vi "Simulate1.vi"() -> ()   [LabVIEW 2014, in "MyHostCode.lvlib"]
uses:
  MyHostCode.lvlib
  FPGACode/Lead Enum.ctl
  <vilib>/Utility/file.llb/Read From Spreadsheet File (DBL).vi
  <vilib>/FPGAPlugInAG/USB-7856R/niLvFpga_Open_USB-7856R.vi
  <vilib>/rvi/interface/common/dynamic/niFpgaDynamicAddResources.vi
  <vilib>/FPGAPlugInAG/Dynamic/niLvFpga_Reset_Dynamic.vi
  <vilib>/FPGAPlugInAG/Dynamic/niLvFpga_Run_Dynamic.vi
  <vilib>/Utility/error.llb/Error Cluster From Error Code.vi
  <vilib>/rvi/errors/niLvFpgaAdjustHostInterfaceError.vi
  <vilib>/FPGAPlugInAG/Dynamic/niLvFpga_Close_Dynamic.vi
  <vilib>/rvi/interface/nirviOpenFPGA/nirviOpenFPGA.xnode
  FPGA Bitfiles/ECGPWMAdaptiveFi_FPGATarget2_ECGAFsim_UMxt-cFiVhs.lvbitx
  <vilib>/rvi/interface/nirviMethod/nirviMethod.xnode
  <vilib>/rvi/interface/nirviReadWriteControl/nirviReadWriteControl.xnode
  <vilib>/rvi/interface/nirviCloseFPGA/nirviCloseFPGA.xnode
  <vilib>/rvi/errors/niLvFpgaMergeErrorWithErrorCode.vi
  <vilib>/FPGAPlugInAG/Dynamic/niLvFpga_StartFifo_Dynamic.vi
  <vilib>/FPGAPlugInAG/Dynamic/niLvFpga_ReadFifo_Dynamic.vi
  <vilib>/rvi/interface/Simulation/niFpgaSimulationCallBeginRW.vi
  NiFpgaLv.dll
  <vilib>/FPGAPlugInAG/Dynamic/niLvFpga_WriteFifo_Dynamic.vi
panel:
  out "Waveform Chart":dbl[](graph)
  out "Waveform Graph 2":dbl[](graph)
  out "Waveform Graph":dbl[](graph)
  out "Data":fxp<+/-,32,16>[](array[numeric]) format="%.21g"
  out "Number":u32
  out "# elements in queue 2":i32
  in  "Reset":bool
  in  "stop":bool
  out "WeightSum":fxp<+/-,33,19> format="%.20g"
  out "BetaProduct":fxp<+/-,32,-1> format="%.33g"
  in  "Rescale":bool
  in  "Decimate":bool
  out "ECG":i16[][](graph)
  out "Gradients":i16[][](graph)
  out "Invasive Blood Pressure":i16[][](graph)
  in  "Plot Info":T2={"Element"={"Lead"=enum."RA", "Filter"=TRUE}, "Element 2"={"Lead"=enum."LA", "Filter"=TRUE}, "Element 3"={"Lead"=enum."LL", "Filter"=TRUE}, "Element 4"={"Lead"=enum."V1", "Filter"=TRUE}, "Element 5"={"Lead"=enum."V2", "Filter"=TRUE}, "Element 6"={"Lead"=enum."V3", "Filter"=TRUE}, "Element 7"={"Lead"=enum."I", "Filter"=TRUE}, "Element 8"={"Lead"=enum."II", "Filter"=TRUE}}
  out "# elements in queue":i32
  in  "File Path Control":path=path "C:/Users/pursley/Documents/Projects/NHLBI/Lederman/Testing/2014-03-21/FL1.txt"
  in  "Beta":fxp<+/-,32,-16>
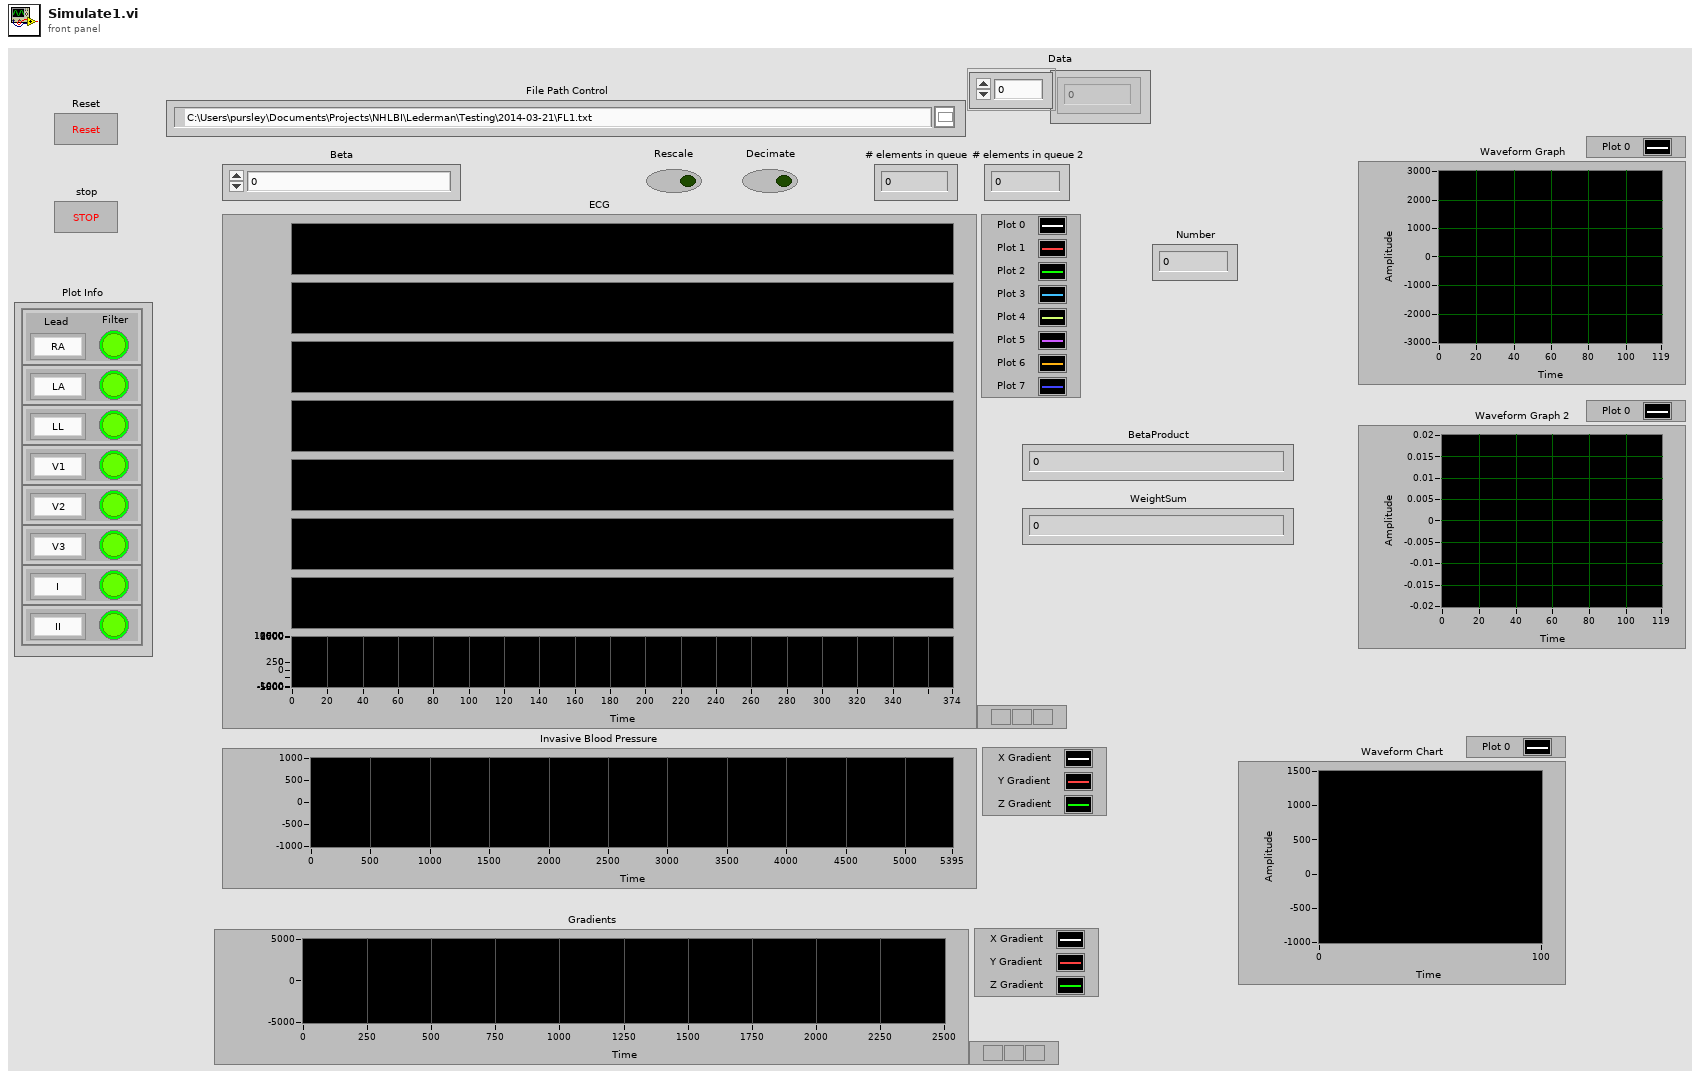
[diagram p1: front panel]
types:
  T1 = typedef "Lead Enum.ctl" = enum16{"RA", "LA", "LL", "V1", "V2", "V3", "V4", "V5", "V6", "I", "II", "III", "aVR", "aVL", "aVF", "Vw"}
  T2 = cluster{"Element":cluster{"Lead":T1, "Filter":bool}, "Element 2":cluster{"Lead":T1, "Filter":bool}, "Element 3":cluster{"Lead":T1, "Filter":bool}, "Element 4":cluster{"Lead":T1, "Filter":bool}, "Element 5":cluster{"Lead":T1, "Filter":bool}, "Element 6":cluster{"Lead":T1, "Filter":bool}, "Element 7":cluster{"Lead":T1, "Filter":bool}, "Element 8":cluster{"Lead":T1, "Filter":bool}}
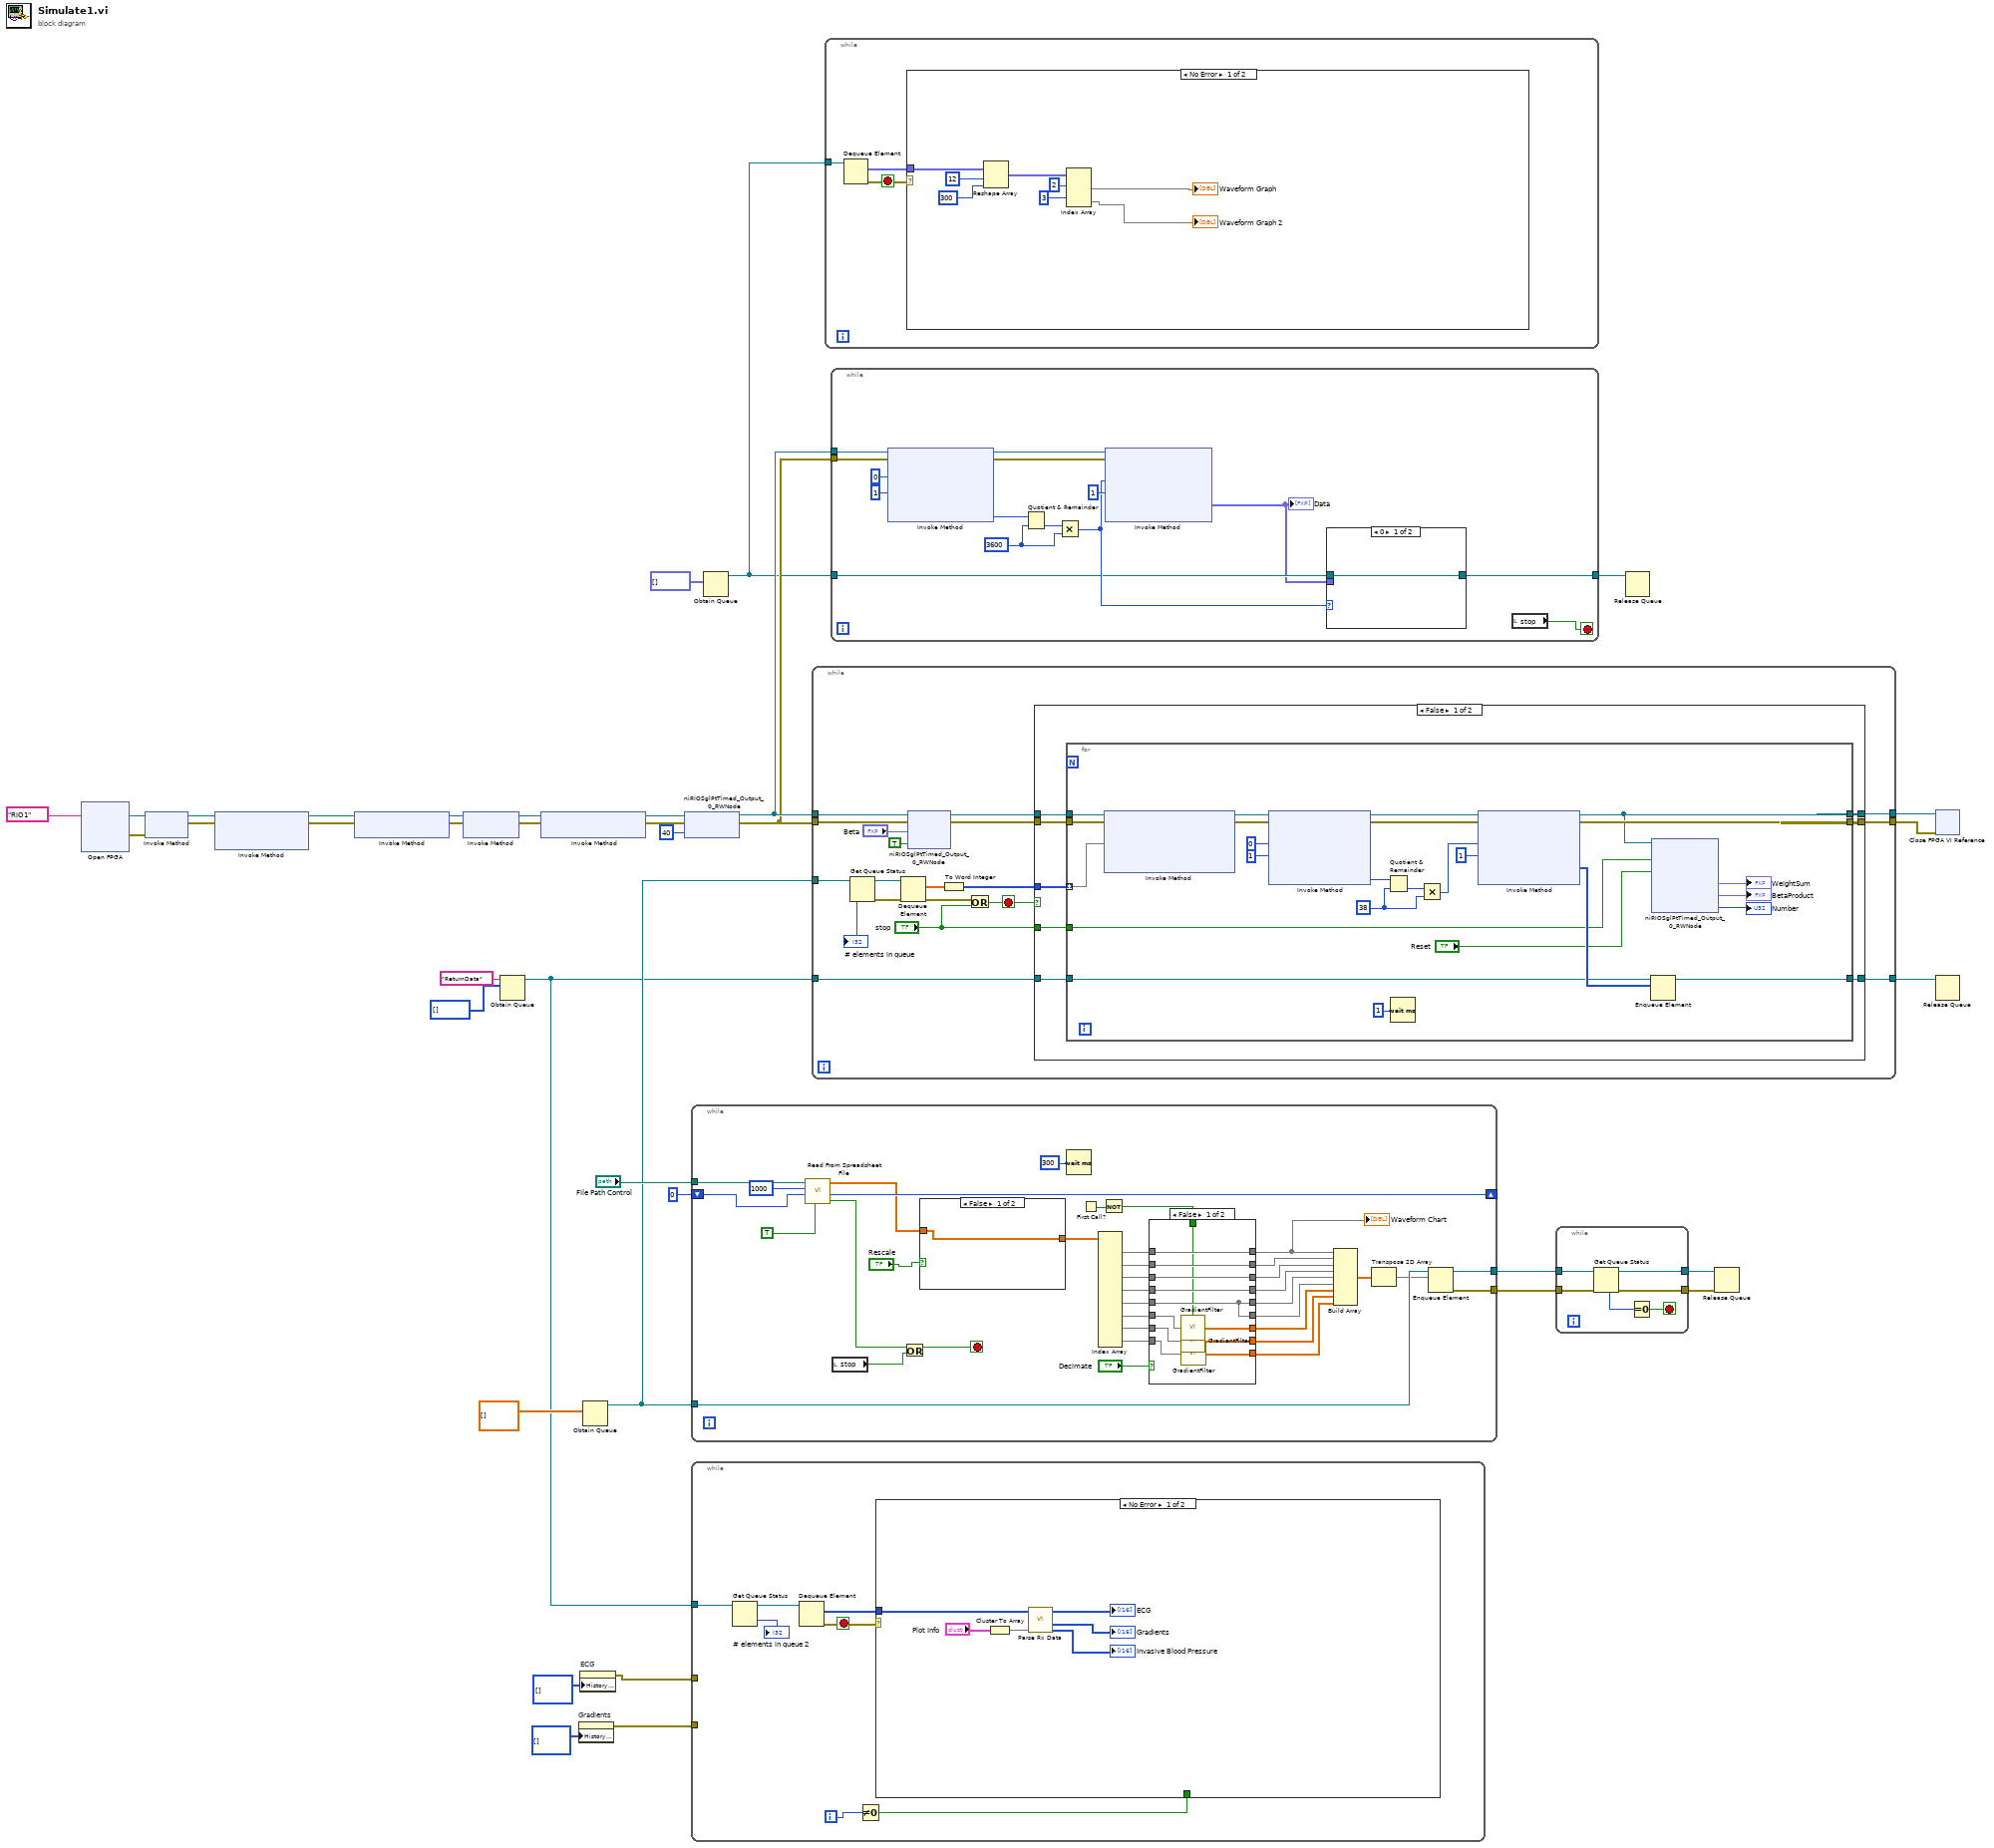
[diagram p0: block diagram]
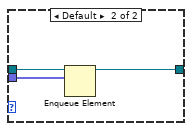
[diagram p3: hidden frame]
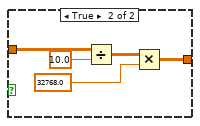
[diagram p5: hidden frame]
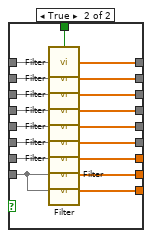
[diagram p6: hidden frame]
diagram:
  n1 = xnode ("Open FPGA")("resource name"=tag "RIO1") -> ("FPGA VI Reference Out"=w37:refnum<k20>, "error out"=w11:errorcluster)  [unwired: 1 in]
  n2 = xnode ("Invoke Method")("FPGA VI Reference In"=w37, "error in"=w11) -> ("FPGA VI Reference Out"=w36:refnum<k20>, "error out"=w35:errorcluster)
  n3 = xnode ("Invoke Method")("FPGA VI Reference In"=w36, "error in"=w35) -> ("FPGA VI Reference Out"=w26:refnum<k20>, "error out"=w25:errorcluster)  [unwired: 1 in]
  n4 = xnode "Invoke Method"("FPGA VI Reference In"=w26, "error in"=w25) -> ("FPGA VI Reference Out"=w14:refnum<k20>, "error out"=w13:errorcluster)
  n5 = xnode "Invoke Method"("FPGA VI Reference In"=w14, "error in"=w13) -> ("FPGA VI Reference Out"=w7:refnum<k20>, "error out"=w6:errorcluster)
  n6 = Obtain Queue(name (unnamed)="ReturnData", element data type=i16[] []) -> (queue out=w19:refnum<queue>)  [unwired: 3 in, 2 out]
  n7 = xnode "Invoke Method"("FPGA VI Reference In"=w7, "error in"=w6) -> ("FPGA VI Reference Out"=w5:refnum<k20>, "error out"=w4:errorcluster)
  n8 = property on="Gradients" class="WFChart (strict)"("History Data"=i16[][] []) -> (error out=w15:errorcluster)  [unwired: 2 in, 1 out]
  n9 = property on="ECG" class="WFChart (strict)"("History Data"=i16[][] []) -> (error out=w16:errorcluster)  [unwired: 2 in, 1 out]
  n10 = Obtain Queue(element data type=dbl[][] [] ("History Data")) -> (queue out=w27:refnum<queue>)  [unwired: 4 in, 2 out]
  n11 = xnode ("niRIOSglPtTimed_Output_0_RWNode")("FPGA VI Reference In"=w5, "error in"=w4, "Filter Size"=i16 40) -> ("FPGA VI Reference Out"=w9:refnum<k20>, "error out"=w8:errorcluster)
  n12 = while {
    tunnel: "File Path Control" -> [w74]
    shift-right: [w72] -> _
    shift-left: 0 ("mark after read (chars.)") -> [w71]
    tunnel: w27 -> [w48]
    tunnel: [w47] -> w31
    tunnel: [w43] -> w33
    stop <- w40 stop-if-true
    n13 = call-poly <vilib>:"Read From Spreadsheet File.vi"("transpose (no:F)"=TRUE, "start of read offset (chars.:0)"=w71, "number of rows (all:-1)"=1000, "file path (dialog if empty)"=w74) -> ("EOF?"=w69:bool, "mark after read (chars.)"=w72:i32, "all rows"=w68:dbl[][])  [unwired: 3 in, 2 out]
    n14 = local read "stop"() -> (w39:bool)
    n15 = Or(x=w69, y=w39) -> (x .or. y?=w40:bool)
    n16 = case shown="False" "Rescale" {
      tunnel: w68 -> [w75 w80]
      tunnel: [w75 w76] -> w67
      frame False {
      }
      frame True {
        n17 = Divide(x=w80, y=10.0) -> (x/y=w78:dbl[][])
        n18 = Multiply(x=w78, y=32768.0) -> (x*y=w76:dbl[][])
      }
    }
    n19 = Wait (ms)(milliseconds to wait=u32 300) -> ()  [unwired: 1 out]
    n20 = First Call?() -> (First Call?: T/F=w65:bool)
    n21 = Index Array(array=w67) -> (element #1=w66:dbl[], element #2=w64:dbl[], element #3=w63:dbl[], element #4=w62:dbl[], element #5=w61:dbl[], element #6=w60:dbl[], element #7=w59:dbl[], element #8=w58:dbl[])  [unwired: 16 in]
    n22 = Not(x=w65) -> (.not. x?=w57:bool)
    n23 = case shown="False" "Decimate" {
      tunnel: w66 -> [w92 w110]
      tunnel: w64 -> [w91 w109]
      tunnel: w63 -> [w90 w108]
      tunnel: w62 -> [w89 w107]
      tunnel: w61 -> [w85 w106]
      tunnel: w60 -> [w86 w105]
      tunnel: w59 -> [w87 w104]
      tunnel: w58 -> [w88 w93]
      tunnel: w57 -> [w81 w103]
      tunnel: [w92 w102] -> w38
      tunnel: [w91 w101] -> w56
      tunnel: [w90 w100] -> w55
      tunnel: [w89 w99] -> w54
      tunnel: [w85 w98] -> w53
      tunnel: [w85 w97] -> w52
      tunnel: [w84 w96] -> w51
      tunnel: [w83 w95] -> w50
      tunnel: [w82 w94] -> w49
      frame False {
        n24 = call "GradientFilter.vi"("Array"=w86, "init/cont (init:F)"=w81) -> ("Decimated Array"=w84:dbl[])
        n25 = call "GradientFilter.vi"("Array"=w87, "init/cont (init:F)"=w81) -> ("Decimated Array"=w83:dbl[])
        n26 = call "GradientFilter.vi"("Array"=w88, "init/cont (init:F)"=w81) -> ("Decimated Array"=w82:dbl[])
      }
      frame True {
        n27 = call "Filter.vi"("Array"=w110, "init/cont (init:F)"=w103) -> ("Decimated Array"=w102:dbl[])
        n28 = call "Filter.vi"("Array"=w109, "init/cont (init:F)"=w103) -> ("Decimated Array"=w101:dbl[])
        n29 = call "Filter.vi"("Array"=w108, "init/cont (init:F)"=w103) -> ("Decimated Array"=w100:dbl[])
        n30 = call "Filter.vi"("Array"=w107, "init/cont (init:F)"=w103) -> ("Decimated Array"=w99:dbl[])
        n31 = call "Filter.vi"("Array"=w106, "init/cont (init:F)"=w103) -> ("Decimated Array"=w98:dbl[])
        n32 = call "Filter.vi"("Array"=w105, "init/cont (init:F)"=w103) -> ("Decimated Array"=w97:dbl[])
        n33 = call "Filter.vi"("Array"=w104, "init/cont (init:F)"=w103) -> ("Decimated Array"=w96:dbl[])
        n34 = call "Filter.vi"("Array"=w93, "init/cont (init:F)"=w103) -> ("Decimated Array"=w95:dbl[])
        n35 = call "Filter.vi"("Array"=w93, "init/cont (init:F)"=w103) -> ("Decimated Array"=w94:dbl[])
      }
    }
    "Waveform Chart" <- w38
    n36 = Build Array(w38, w56, w55, w54, w53, w52, w51, w50, w49) -> (w46:dbl[][])
    n37 = Transpose 2D Array(2D array=w46) -> (transposed array=w45:dbl[][])
    n38 = Enqueue Element(queue=w48, element=w45) -> (queue out=w47:refnum<queue>, error out=w43:errorcluster)  [unwired: 2 in, 1 out]
  }
  n39 = while {
    tunnel: w19 -> [w117]
    tunnel: w16 -> [_]
    tunnel: w15 -> [_]
    i -> [w114]
    stop <- w116 stop-if-true
    n40 = Get Queue Status(queue=w117) -> (queue out=w112:refnum<queue>, # elements in queue=→"# elements in queue 2":i32)  [unwired: 2 in, 6 out]
    n41 = Dequeue Element(queue=w112) -> (element=w115:i16[], error out=w116:errorcluster)  [unwired: 2 in, 2 out]
    n42 = Not Equal To 0?(x=w114) -> (x != 0?=w113:bool)
    n43 = case shown="No Error" w116 {
      tunnel: w115 -> [w122 _]
      tunnel: w113 -> [_ _]
      frame No Error {
        n44 = Cluster To Array(cluster="Plot Info") -> (array=w118:cluster{"Lead":T1, "Filter":bool}[])
        n45 = call "Parse Rx Data.vi"("Plot Info"=w118, "Input Data"=w122) -> ("Pressures"=→"Invasive Blood Pressure":i16[][], "Gradients"=→"Gradients":i16[][], "ECG Data"=→"ECG":i16[][])  [unwired: 6 in, 1 out]
      }
      frame Error {
      }
    }
  }
  n46 = Obtain Queue(element data type=fxp<+/-,32,16>[] [] ("Data")) -> (queue out=w1:refnum<queue>)  [unwired: 4 in, 2 out]
  n47 = while {
    tunnel: w9 -> [w141]
    tunnel: w8 -> [w140]
    tunnel: w27 -> [w136]
    tunnel: w19 -> [w131]
    tunnel: [w130] -> w22
    tunnel: [w129] -> w21
    tunnel: [w128] -> w20
    stop <- w125 stop-if-true
    n48 = Get Queue Status(queue=w136) -> (queue out=w137:refnum<queue>, error out=w139:errorcluster, # elements in queue=→"# elements in queue":i32)  [unwired: 2 in, 5 out]
    n49 = Dequeue Element(queue=w137, error in (no error)=w139) -> (element=w135:dbl[][], error out=w126:errorcluster)  [unwired: 1 in, 2 out]
    n50 = xnode ("niRIOSglPtTimed_Output_0_RWNode")("FPGA VI Reference In"=w141, "error in"=w140, "Beta"="Beta", "Start 0"=TRUE) -> ("FPGA VI Reference Out"=w134:refnum<k20>, "error out"=w133:errorcluster)
    n51 = To Word Integer(number=w135) -> (16bit integer=w132:i16[][])
    n52 = Or(x=w126, y="stop") -> (x .or. y?=w125:bool)
    n53 = case shown="False" w125 {
      tunnel: w132 -> [w150 _]
      tunnel: w134 -> [w149 w177]
      tunnel: w133 -> [w148 w176]
      tunnel: w131 -> [w147 w178]
      tunnel: [w146 w178] -> w130
      tunnel: [w145 w177] -> w129
      tunnel: [w144 w176] -> w128
      tunnel: "stop" -> [w143 _]
      frame False {
        n54 = for {
          tunnel: w150 -> [w173] mode=indexing
          tunnel: w149 -> [w175]
          tunnel: w148 -> [w174]
          tunnel: w147 -> [w160]
          tunnel: [w159] -> w146
          tunnel: [w156] -> w145
          tunnel: [w157] -> w144
          tunnel: w143 -> [w153]
          w171 = u32 38 ("y")
          n55 = xnode "Invoke Method"("FPGA VI Reference In"=w175, "error in"=w174, "Data"=w173) -> ("FPGA VI Reference Out"=w163:refnum<k20>, "error out"=w162:errorcluster)  [unwired: 1 in, 1 out]
          n56 = xnode "Invoke Method"("FPGA VI Reference In"=w163, "error in"=w162, "Number of Elements"=u32 0, "Timeout (ms)"=1) -> ("FPGA VI Reference Out"=w166:refnum<k20>, "error out"=w167:errorcluster, "Elements Remaining"=w168:u32)  [unwired: 1 out]
          n57 = Quotient & Remainder(x=w168, y=w171) -> (floor(x/y)=w170:u32)  [unwired: 1 out]
          n58 = Wait (ms)(milliseconds to wait=u32 1) -> ()  [unwired: 1 out]
          n59 = Multiply(x=w170, y=w171) -> (x*y=w172:u32)
          n60 = xnode "Invoke Method"("FPGA VI Reference In"=w166, "error in"=w167, "Number of Elements"=w172, "Timeout (ms)"=1) -> ("FPGA VI Reference Out"=w156:refnum<k20>, "error out"=w157:errorcluster, "Data"=w161:i16[])  [unwired: 1 out]
          n61 = Enqueue Element(queue=w160, element=w161) -> (queue out=w159:refnum<queue>)  [unwired: 2 in, 2 out]
          n62 = xnode ("niRIOSglPtTimed_Output_0_RWNode")("FPGA VI Reference In"=w156, "stop"=w153, "Reset"="Reset") -> ("WeightSum"=→"WeightSum":fxp<+/-,33,19>, "BetaProduct"=→"BetaProduct":fxp<+/-,32,-1>, "Number"=→"Number":u32)  [unwired: 1 in, 2 out]
        }
      }
      frame True {
      }
    }
  }
  n63 = while {
    tunnel: w1 -> [w181]
    stop <- w179 stop-if-true
    n64 = Dequeue Element(queue=w181) -> (element=w180:fxp<+/-,32,16>[], error out=w179:errorcluster)  [unwired: 2 in, 2 out]
    n65 = case shown="No Error" w179 {
      tunnel: w180 -> [w189 _]
      frame No Error {
        n66 = Reshape Array(w189, 12 ("dimension size"), 300 ("dimension size")) -> (w185:fxp<+/-,32,16>[][])
        n67 = Index Array(array=w185, index (row) #1=2 ("index (row)"), index (row) #2=3 ("index (row)")) -> (element #1=→"Waveform Graph":fxp<+/-,32,16>[], element #2=→"Waveform Graph 2":fxp<+/-,32,16>[])  [unwired: 2 in]
      }
      frame Error {
      }
    }
  }
  n68 = while {
    tunnel: w9 -> [w204]
    tunnel: w8 -> [w203]
    tunnel: w1 -> [w192]
    tunnel: [w190] -> w2
    stop <- w195 stop-if-true
    w197 = u32 3600 ("y")
    n69 = xnode "Invoke Method"("FPGA VI Reference In"=w204, "error in"=w203, "Number of Elements"=u32 0, "Timeout (ms)"=1) -> ("FPGA VI Reference Out"=w200:refnum<k20>, "error out"=w199:errorcluster, "Elements Remaining"=w196:u32)  [unwired: 1 out]
    n70 = Quotient & Remainder(x=w196, y=w197) -> (floor(x/y)=w198:u32)  [unwired: 1 out]
    n71 = Multiply(x=w198, y=w197) -> (x*y=w193:u32)
    n72 = xnode "Invoke Method"("FPGA VI Reference In"=w200, "error in"=w199, "Number of Elements"=w193, "Timeout (ms)"=1) -> ("Data"=w191:fxp<+/-,32,16>[])  [unwired: 3 out]
    "Data" <- w191
    n73 = case shown="0" w193 {
      tunnel: w192 -> [w205 w208]
      tunnel: w191 -> [_ w207]
      tunnel: [w205 w206] -> w190
      frame 0 {
      }
      frame Default {
        n74 = Enqueue Element(queue=w208, element=w207) -> (queue out=w206:refnum<queue>)  [unwired: 2 in, 2 out]
      }
    }
    n75 = local read "stop"() -> (w195:bool)
  }
  n76 = while {
    tunnel: w31 -> [w214]
    tunnel: [w213] -> w32
    tunnel: w33 -> [w212]
    tunnel: [w211] -> w34
    stop <- w209 stop-if-true
    n77 = Get Queue Status(queue=w214, error in (no error)=w212) -> (queue out=w213:refnum<queue>, error out=w211:errorcluster, # elements in queue=w210:i32)  [unwired: 1 in, 5 out]
    n78 = Equal To 0?(x=w210) -> (x = 0?=w209:bool)
  }
  n79 = Release Queue(queue=w2) -> ()  [unwired: 2 in, 3 out]
  n80 = Release Queue(queue=w32, error in (no error)=w34) -> ()  [unwired: 1 in, 3 out]
  n81 = xnode ("Close FPGA VI Reference")("FPGA VI Reference In"=w21, "error in"=w20) -> ()  [unwired: 1 out]
  n82 = Release Queue(queue=w22) -> ()  [unwired: 2 in, 3 out]
